vi "DrawLine.vi"(6 "yEnd":i16, 7 "xEnd":i16, 9 "yStart":i16, 10 "xStart":i16, 11 "PictureIn":picture) -> (3 "PictureOut":picture)   [LabVIEW 2014]
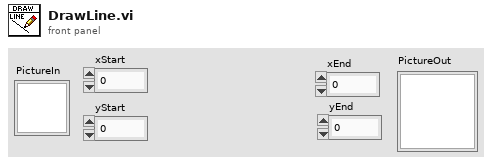
[diagram p1: front panel]
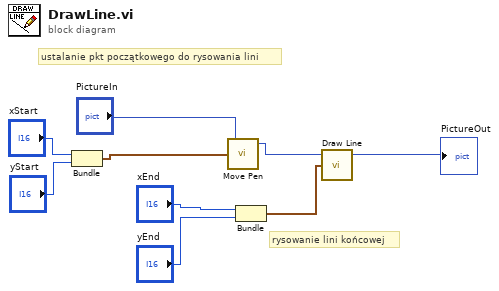
[diagram p0: block diagram]
diagram:
  # "rysowanie lini końcowej"
  # "ustalanie pkt początkowego do rysowania lini"
  n1 = Bundle("xStart"="xStart", "yStart"="yStart") -> (w7:cluster{"xStart":i16, "yStart":i16})  [unwired: 1 in]
  n2 = call <vilib>:"Move Pen.vi"("new position"=w7, "picture"="PictureIn") -> ("new picture"=w5:picture)  [unwired: 3 in]
  n3 = Bundle("xEnd"="xEnd", "yEnd"="yEnd") -> (w1:cluster{"xEnd":i16, "yEnd":i16})  [unwired: 1 in]
  n4 = call <vilib>:"Draw Line.vi"("picture"=w5, "end point"=w1) -> ("new picture"=→"PictureOut":picture)  [unwired: 7 in]
